vi "TextFit_Count Pixel Width.vi"(8 "Error":errorcluster, 11 "Counter Array":T1[](array[typedef])) -> (0 "Error Out":errorcluster, 3 "Pixel Width Out":i32)   [LabVIEW 2014]
doc: "Counts the amount of pixels the character array will use"
uses:
  Controls/Cluster/Cluster_Character Size and Priority Data.ctl
  Controls/String_Picture/String Char Normal.ctl
  Controls/Enum/ENUM_Font Size Select.ctl
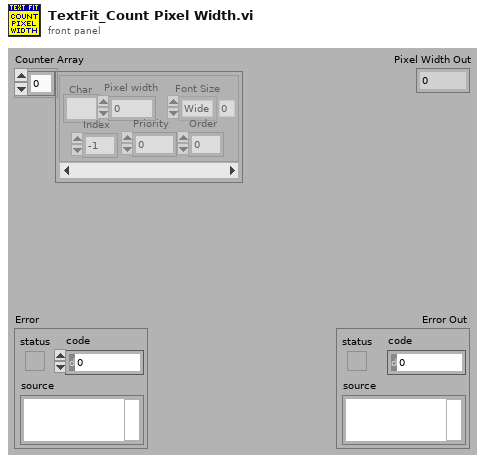
[diagram p1: front panel]
types:
  T1 = typedef "Cluster_Character Size and Priority Data.ctl" = cluster{"Char":T2, "Font Size":T3, "Pixel width":i32, "Priority":i32, "Order":i32, "Index":i32}
  T2 = typedef "String Char Normal.ctl" = string
  T3 = typedef "ENUM_Font Size Select.ctl" = enum16{"Wide", "Med", "Thin"}
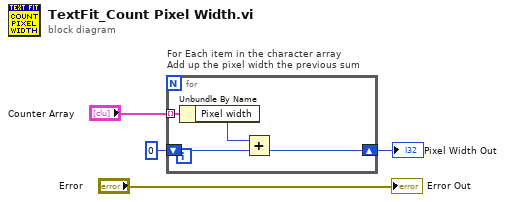
[diagram p0: block diagram]
diagram:
  n1 = for "For Each item in the character array\nAdd up the pixel width the previous sum" {
    tunnel: "Counter Array" -> [w8] mode=indexing
    shift-right: [w5] -> w4
    shift-left: 0 -> [w6]
    n2 = Unbundle By Name(w8) -> ("Pixel width"=w7:i32)
    n3 = Add(x=w7, y=w6) -> (x+y=w5:i32)
  }
  "Pixel Width Out" <- w4
  "Error Out" <- "Error"
